vi "AutoWait.vi"(11 "BrickReference in":T1) -> (0 "TimeDelay":u32, 3 "BrickReference out":T1)   [LabVIEW 2012, in "BlockParty4150.lvrbt"]
uses:
  BlockParty4150.lvrbt
  <vilib>/NXT/Subs/LVHSConnector.ctl
  <vilib>/NXT/LegoClasses/BrickReference/BrickReference.lvclass
  <vilib>/NXT/Block Support/NXT_ButtonSelector.ctl
  <vilib>/NXT/Dual Mode Library/prims/inRangeAndCoerce/inRangeAndCoerce_int.vi
  <vilib>/NXT/Dual Mode Library/Display/drawNumber.vi
  <vilib>/NXT/Dual Mode Library/Sound/Tone.vi
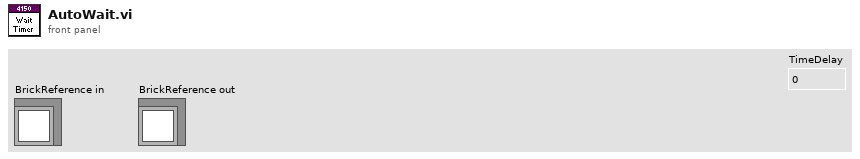
[diagram p1: front panel]
types:
  T1 = typedef "LVHSConnector.ctl" = refnum<class "BrickReference.lvclass">
  T2 = typedef "NXT_ButtonSelector.ctl" = u16
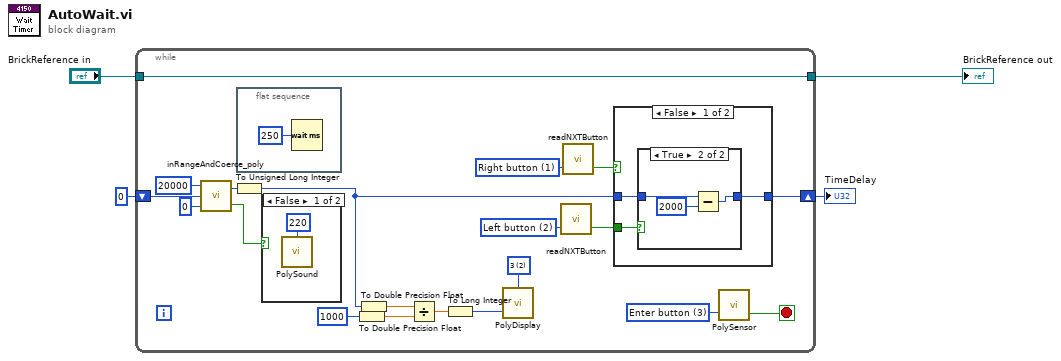
[diagram p0: block diagram]
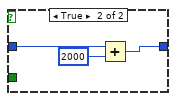
[diagram p4: hidden frame]
diagram:
  n1 = while {
    tunnel: [w24] -> w1
    tunnel: "BrickReference in" -> [w24]
    shift-right: [w17] -> w2
    shift-left: u32 0 ("Power/Speed 1") -> [w10]
    stop <- w22 stop-if-true
    w16 = i16 2 items=["1", "2", "3", "4", "5", "6", "7", "8"] ("Line")
    w19 = T2 1 items=["Enter button"=3, "Left button"=2, "Right button"=1] ("Button (Enter button)")
    w18 = T2 2 items=["Enter button"=3, "Left button"=2, "Right button"=1] ("Button (Enter button)")
    w23 = T2 3 items=["Enter button"=3, "Left button"=2, "Right button"=1] ("Button (Enter button)")
    n2 = call-poly <vilib>:"inRangeAndCoerce_poly.vi"("lower limit"=0, "x"=w10, "upper limit"=20000) -> ("In Range?"=w5:bool, "coerced(x)"=w7:i32)
    n3 = To Unsigned Long Integer(number=w7) -> (unsigned 32bit integer=w6:u32)
    n4 = flat-sequence {
      frame #0 {
        n5 = Wait (ms)(milliseconds to wait=u32 250) -> ()  [unwired: 1 out]
      }
    }
    n6 = case shown="False" w5 {
      frame False {
        n7 = call-poly <vilib>:"PolySound.vi"("Tone (440 Hz)"=u16 220) -> ()  [unwired: 3 in, 1 out]
      }
      frame True {
      }
    }
    n8 = To Double Precision Float(number=u32 1000 ("Power/Speed 1")) -> (double precision float=w11:dbl)
    n9 = To Double Precision Float(number=w6) -> (double precision float=w13:dbl)
    n10 = Divide(x=w13, y=w11) -> (x/y=w14:dbl)
    n11 = To Long Integer(number=w14) -> (32bit integer=w12:i32)
    n12 = call-poly <vilib>:"PolyDisplay.vi"("number"=w12, "Line"=w16) -> ()  [unwired: 2 in, 1 out]
    n13 = call <vilib>:"readNXTButton.vi"("Button (Enter button)"=w18) -> ("Yes/No"=w21:bool)  [unwired: 2 in, 1 out]
    n14 = call <vilib>:"readNXTButton.vi"("Button (Enter button)"=w19) -> ("Yes/No"=w20:bool)  [unwired: 2 in, 1 out]
    n15 = case shown="False" w20 {
      tunnel: w21 -> [w29 _]
      tunnel: [w28 w35] -> w17
      tunnel: w6 -> [w27 w36]
      frame False {
        n16 = case shown="True" w29 {
          tunnel: [w30 w32] -> w28
          tunnel: w27 -> [w30 w33]
          frame False {
          }
          frame True {
            n17 = Subtract(x=w33, y=u32 2000) -> (x-y=w32:u32)
          }
        }
      }
      frame True {
        n18 = Add(x=w36, y=u32 2000) -> (x+y=w35:u32)
      }
    }
    n19 = call-poly <vilib>:"PolySensor.vi"("Button (Enter button)"=w23) -> ("Yes/No"=w22:bool)  [unwired: 2 in, 1 out]
  }
  "BrickReference out" <- w1
  "TimeDelay" <- w2
